vi "BS find buoys demo.vi"() -> ()   [LabVIEW 2012]
uses:
  <vilib>/vision/NI_Vision_Development_Module.lvlib
panel:
  out "Buoy location string":string
  out "Buoy Array":cluster{i16, i16}[](array[cluster])
  out "found?":bool
  in  "Image file name":string="boats and buoys.bmp"
  in  "stop":bool
  out "error out":errorcluster
  out "Working Image":T1(plugin-control)
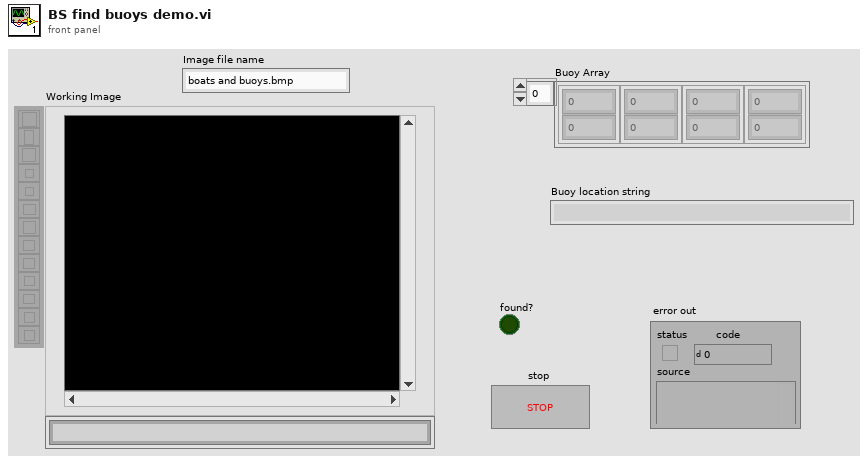
[diagram p1: front panel]
types:
  T1 = typedef "IMAQ Image.ctl" = refnum<image>
  T2 = enum32{"AutoM", "Close", "Dilate", "Erode", "Gradient", "Gradient in", "Gradient out", "HitMiss", "Open", "PClose", "POpen", "Thick", "Thin"}
  T3 = typedef "Image Type" = u32
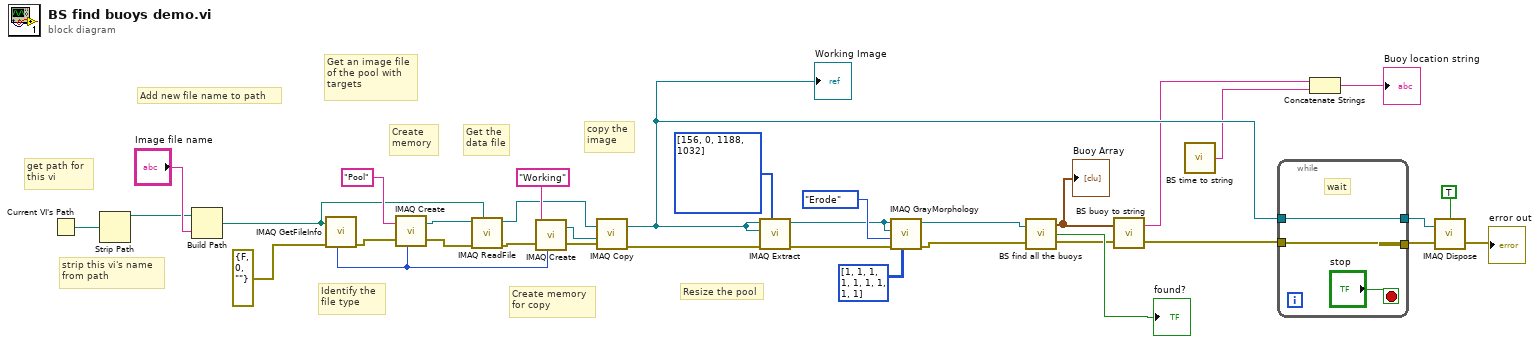
[diagram p0: block diagram]
diagram:
  # "Resize the pool"
  # "Create memory\nfor copy"
  # "copy the\nimage"
  # "Add new file name to path"
  # "strip this vi's name \nfrom path"
  # "get path for \nthis vi"
  # "Get the \ndata file"
  # "Create \nmemory"
  # "Identify the \nfile type"
  # "Get an image file\nof the pool with\ntargets"
  n1 = Current VI's Path() -> (path=w26:path)
  n2 = Strip Path(path=w26) -> (stripped path=w25:path)  [unwired: 1 out]
  n3 = Build Path(base path=w25, name or relative path="Image file name") -> (appended path=w24:path)
  n4 = call "IMAQ GetFileInfo"("error in (no error)"=errorcluster {"status"=FALSE, "code"=0, "source"=""}, "File Path"=w24) -> ("error out"=w35:errorcluster, "Image Type"=w17:T3)  [unwired: 3 in, 5 out]
  n5 = call "IMAQ Create"("Image Name"="Pool", "Image Type"=w17, "error in (no error)"=w35) -> ("New Image"=w33:T1, "error out"=w30:errorcluster)  [unwired: 2 in]
  n6 = call "IMAQ ReadFile"("File Path"=w24, "error in (no error)"=w30, "Image"=w33) -> ("error out"=w18:errorcluster, "Image Out"=w19:T1)  [unwired: 4 in, 3 out]
  n7 = call "IMAQ Create"("Image Name"="Working", "Image Type"=w17, "error in (no error)"=w18) -> ("New Image"=w28:T1, "error out"=w31:errorcluster)  [unwired: 2 in]
  n8 = call "IMAQ Copy"("error in (no error)"=w31, "Image Dst"=w28, "Image Src"=w19) -> ("error out"=w15:errorcluster, "Image Dst Out"=w14:T1)  [unwired: 3 in]
  "Working Image" <- w14
  n9 = call "IMAQ Extract"("Optional Rectangle"=i32[] [156, 0, 1188, 1032], "error in (no error)"=w15, "Image Dst"=w14, "Image Src"=w14) -> ("error out"=w11:errorcluster, "Image Dst Out"=w10:T1)  [unwired: 6 in]
  n10 = call "IMAQ GrayMorphology"("Structuring Element"=i32[][] [[1, 1, 1], [1, 1, 1], [1, 1, 1]] ("Structuring Element (Gray Morphology 1)"), "error in (no error)"=w11, "Operation"=T2."Erode" ("Operation (Gray Morphology 1)"), "Image Dst"=w10, "Image Src"=w10) -> ("error out"=w8:errorcluster, "Image Dst Out"=w9:T1)  [unwired: 2 in, 3 out]
  n11 = call "BS find all the buoys.vi"("Image Src"=w9, "error in"=w8) -> ("Buoy Array"=w6:cluster{i16, i16}[], "Buoys found?"=→"found?":bool, "error out"=w5:errorcluster)
  "Buoy Array" <- w6
  n12 = call "BS buoy to string.vi"("error in"=w5, "Buoy Array"=w6) -> ("error out"=w4:errorcluster, "Buoy location string"=w3:string)
  n13 = call "BS time to string.vi"() -> ("time string"=w2:string)  [unwired: 1 in]
  n14 = while {
    tunnel: w14 -> [w36]
    tunnel: w4 -> [w37]
    tunnel: [w37] -> w23
    tunnel: [w36] -> w21
    stop <- "stop" stop-if-true
    # "wait"
  }
  n15 = Concatenate Strings(w3, w2) -> (→"Buoy location string":string)
  n16 = call "IMAQ Dispose"("All Images? (No)"=TRUE, "Image"=w21, "error in (no error)"=w23) -> ("error out"=→"error out":errorcluster)  [unwired: 3 in]
